vi "SiosIfmGetDeviceInfoPSDCount.vi"(1 "devNumber":i32) -> (0 "PSD Count":i32)   [LabVIEW 2009]
uses:
  siosifm.dll
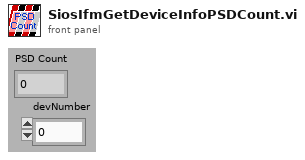
[diagram p1: front panel]
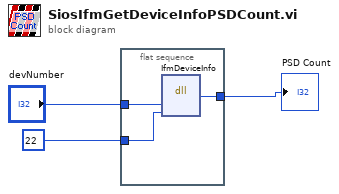
[diagram p0: block diagram]
diagram:
  n1 = flat-sequence {
    tunnel: [w6] -> w1
    tunnel: "devNumber" -> [w5]
    tunnel: 22 ("requestedInfo") -> [w4]
    frame #0 {
      n2 = dll-call lib="C:/WORK/Artem/RE-10/SIOS_IfmDLL/siosifm.dll" fn="IfmDeviceInfo"("devNumber"=w5, "requestedInfo"=w4) -> ("requestedInfo"=w6:i32)  [unwired: 5 in, 2 out]
    }
  }
  "PSD Count" <- w1
